vi "Example.vi"() -> ()   [LabVIEW 2013]
uses:
  BarcodeType.ctl
  EAN-13/EAN-13.lvclass
  Code39/Code39.lvclass
  Code128/Code128.lvclass
  UPC/UPC.lvclass
  Linear Barcode/Linear Barcode.lvclass
  BarCodes.lvlib
panel:
  in  "BarcodeType":T1
  out "Valid Value":bool
  in  "Input":string="123456789012"
  out "Barcode":picture
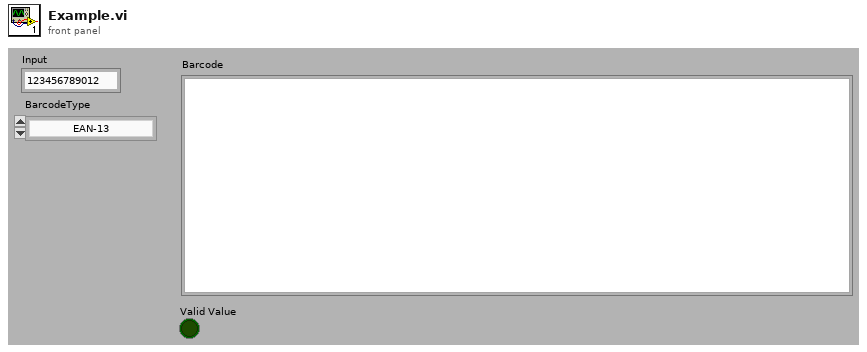
[diagram p1: front panel]
types:
  T1 = typedef "BarCodes.lvlib/BarcodeType.ctl" = enum16{"EAN-13", "UPC", "Code 39 (3 of 9)", "Code 128"}
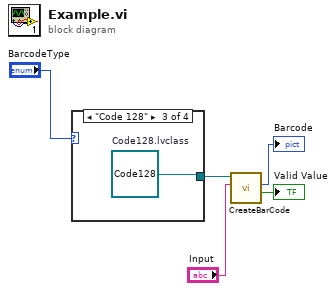
[diagram p0: block diagram]
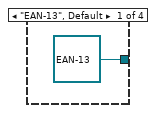
[diagram p2: hidden frame]
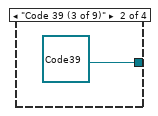
[diagram p3: hidden frame]
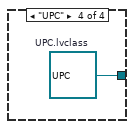
[diagram p4: hidden frame]
diagram:
  n1 = case shown="\"Code 128\"" "BarcodeType" {
    tunnel: [refnum<class "EAN-13.lvclass"> refnum ("EAN-13.lvclass") refnum<class "Code39.lvclass"> refnum ("Code39.lvclass") w8 w9] -> w1
    frame "EAN-13", Default {
    }
    frame "Code 39 (3 of 9)" {
    }
    frame "Code 128" {
      w8 = refnum<class "Code128.lvclass"> refnum  # Code128.lvclass
    }
    frame "UPC" {
      w9 = refnum<class "UPC.lvclass"> refnum  # UPC.lvclass
    }
  }
  n2 = call-dynamic "CreateBarCode.vi"("Input"="Input", "BarCode in"=w1) -> ("Valid Value"=→"Valid Value":bool, "Barcode"=→"Barcode":picture)  [unwired: 6 in, 2 out]
